vi "Queue Reference (library variable).vi"() -> ()   [LabVIEW 2020, in "Error Manager.lvlib" / "Testers.lvlib" / "Anti-Spam Tester.lvlib" / "AST MHL Queue.lvlib"]
uses:
  AST MHL Queue.lvlib
  Command (enum).ctl
  Message (cluster).ctl
panel:
  in  "Queue Reference":refnum<queue>
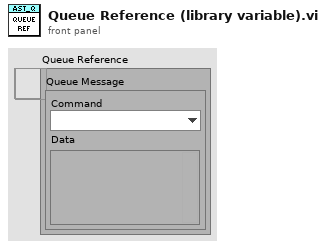
[diagram p1: front panel]
diagram:
